vi "Test Search-Split String.vi"(8 "error in (no error)":errorcluster) -> (0 "error out":errorcluster, 3 "Pass?":bool)   [LabVIEW 2020]
uses:
  G-Unicode/Types/UTF-8 String/UTF-8 String.lvclass/UTF-8 String.ctl
  9ff3dfa9-f8ba-4427-ad5f-a2fde7b6c77a.vi
  850149eb-9a48-45f9-aca9-3728815fdd3d.vi
  d33158b6-7e12-4a86-8fbe-645f2238ccec.vi
  2fcd0a92-766f-4ab9-bfdc-e2927028f498.vi
  451e0aa1-621d-4b4c-868c-abfc6350e238.vi
  77c8659a-ed0f-4c8d-a4b1-7b3f6f0d4640.vi
  G-Unicode/Private/Conversion/String as Encoded String.vi
  G-Unicode/Private/Conversion/Polymorphic VIs/String as Encoded String (LabVIEW String).vi
  G-Unicode/Private/Library/gu_search_split_string.vi
  850149eb-9a48-45f9-aca9-3728815fdd3d.vi/3a31b270-3bb6-4c58-a256-c5fcc2c98f09.vi
  850149eb-9a48-45f9-aca9-3728815fdd3d.vi/0ec5df2d-ef9b-4f84-a6a8-ffcedd45c4dc.vi
  d33158b6-7e12-4a86-8fbe-645f2238ccec.vi/3a31b270-3bb6-4c58-a256-c5fcc2c98f09.vi
  d33158b6-7e12-4a86-8fbe-645f2238ccec.vi/0ec5df2d-ef9b-4f84-a6a8-ffcedd45c4dc.vi
  451e0aa1-621d-4b4c-868c-abfc6350e238.vi/3a31b270-3bb6-4c58-a256-c5fcc2c98f09.vi
  451e0aa1-621d-4b4c-868c-abfc6350e238.vi/0ec5df2d-ef9b-4f84-a6a8-ffcedd45c4dc.vi
  77c8659a-ed0f-4c8d-a4b1-7b3f6f0d4640.vi/3a31b270-3bb6-4c58-a256-c5fcc2c98f09.vi
  77c8659a-ed0f-4c8d-a4b1-7b3f6f0d4640.vi/0ec5df2d-ef9b-4f84-a6a8-ffcedd45c4dc.vi
  G-Unicode/Private/Conversion/Text to UTF-8.vi
  G-Unicode/Private/Conversion/Polymorphic VIs/Text to UTF-8 (LabVIEW String).vi
  G-Unicode/Private/Memory/Copy String.vi
  G-Unicode/Private/Library/Result To Error.vi
  G-Unicode/Private/Conversion/Text as Encoded String.vi
  G-Unicode/Private/Conversion/Polymorphic VIs/Text as Encoded String (LabVIEW String).vi
  G-Unicode/Private/Conversion/Polymorphic VIs/Text as Encoded String (UTF-8 String).vi
  G-Unicode/Private/Memory/Copy String.vi/4d47babd-4a2d-4eb7-b91b-7e707d692665.vi
  G-Unicode/Private/Library/gu_free.vi
  G-Unicode/Types/UTF-8 String/Read Encoded UTF-8 String.vi
  <vilib>/Utility/error.llb/Error Cluster From Error Code.vi
  G-Unicode/Types/UTF-8 String/UTF-8 String.lvclass
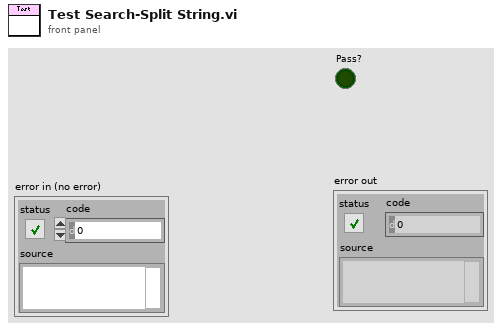
[diagram p1: front panel]
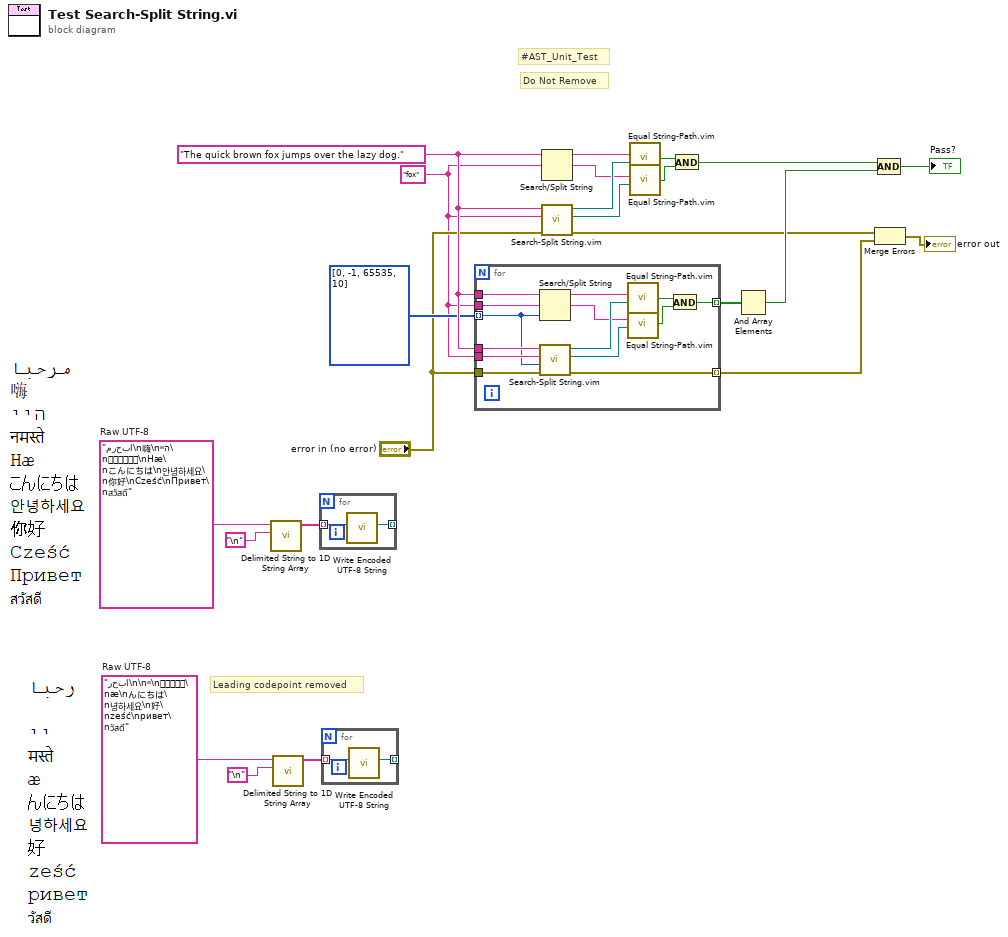
[diagram p0: block diagram]
diagram:
  w1 = "fox" ("search string/char (-)")
  w16 = "رحبا\n\nיי\nमस्ते\næ\nんにちは\n녕하세요\n好\nześć\nривет\nวัสดี"  # Raw UTF-8
  w10 = "The quick brown fox jumps over the lazy dog." ("string")
  w22 = "مرحبا\n嗨\nהיי\nनमस्ते\nHæ\nこんにちは\n안녕하세요\n你好\nCześć\nПривет\nสวัสดี"  # Raw UTF-8
  # "Leading codepoint removed"
  # "Do Not Remove"
  # "#AST_Unit_Test"
  n1 = call <vilib>:"Delimited String to 1D String Array.vi"("delimiter"="\n", "delimited string"=w22) -> ("string array"=w21:string[])  [unwired: 9 in]
  n2 = call <vilib>:"Delimited String to 1D String Array.vi"("delimiter"="\n", "delimited string"=w16) -> ("string array"=w17:string[])  [unwired: 9 in]
  n3 = for {
    tunnel: w21 -> [w25] mode=indexing
    tunnel: [w24] -> _ mode=indexing
    n4 = call "Write Encoded UTF-8 String.vi"("Encoded UTF-8 String"=w25) -> ("UTF-8 String"=w24:refnum<class "UTF-8 String.lvclass">)  [unwired: 10 in]
  }
  n5 = for {
    tunnel: w17 -> [w27] mode=indexing
    tunnel: [w26] -> _ mode=indexing
    n6 = call "Write Encoded UTF-8 String.vi"("Encoded UTF-8 String"=w27) -> ("UTF-8 String"=w26:refnum<class "UTF-8 String.lvclass">)  [unwired: 10 in]
  }
  n7 = for {
    tunnel: [w37] -> w8 mode=indexing
    tunnel: w10 -> [w36]
    tunnel: w1 -> [w35]
    tunnel: w10 -> [w34]
    tunnel: w1 -> [w33]
    tunnel: "error in (no error)" -> [w32]
    tunnel: [w30] -> w9 mode=indexing
    tunnel: i32[] [0, -1, 65535, 10] -> [w28] mode=indexing
    n8 = Search/Split String(string=w36, search string/char (-)=w35, offset (0)=w28) -> (substring before match=w31:string, match + rest of string=w29:string)  [unwired: 1 out]
    n9 = call "Search-Split String.vim"("error in"=w32, "Offset (0)"=w28, "Search String/Codepoint"=w33, "String"=w34) -> ("error out"=w30:errorcluster, "Match + Rest Of String"=w39:refnum<class "UTF-8 String.lvclass">, "Substring Before Match"=w38:refnum<class "UTF-8 String.lvclass">)  [unwired: 5 in]
    n10 = call "Equal String-Path.vim"("y"=w38, "x"=w31) -> ("Equal?"=w40:bool)  [unwired: 7 in, 1 out]
    n11 = call "Equal String-Path.vim"("y"=w39, "x"=w29) -> ("Equal?"=w41:bool)  [unwired: 7 in, 1 out]
    n12 = And(x=w40, y=w41) -> (x .and. y?=w37:bool)
  }
  n13 = Search/Split String(string=w10, search string/char (-)=w1) -> (substring before match=w5:string, match + rest of string=w3:string)  [unwired: 1 in, 1 out]
  n14 = call "Search-Split String.vim"("error in"="error in (no error)", "Search String/Codepoint"=w1, "String"=w10) -> ("error out"=w4:errorcluster, "Match + Rest Of String"=w14:refnum<class "UTF-8 String.lvclass">, "Substring Before Match"=w19:refnum<class "UTF-8 String.lvclass">)  [unwired: 6 in]
  n15 = call "Equal String-Path.vim"("y"=w19, "x"=w5) -> ("Equal?"=w13:bool)  [unwired: 7 in, 1 out]
  n16 = call "Equal String-Path.vim"("y"=w14, "x"=w3) -> ("Equal?"=w12:bool)  [unwired: 7 in, 1 out]
  n17 = And(x=w13, y=w12) -> (x .and. y?=w11:bool)
  n18 = And Array Elements(Boolean array=w8) -> (logical AND=w7:bool)
  n19 = Merge Errors(w4, w9) -> (→"error out":errorcluster)
  n20 = Compound Arithmetic op=AND(w11, w7) -> (→"Pass?":bool)
